vi "SParam VST Init.vi"(8 "error in":errorcluster, 11 "SPML Settings":T2={"VST Resource Name"="VNA-5633", "RFSG Port"="", "RFmx Port"="", "RF Out Switch"="VNA-5633", "RF Out Connection"={"Common RFout"="", "Port1 Incident"="", "Port2 Incident"=""}, "RF In Switch"="VNA-5633", "RF In Connection"={"Common RFin"="", "Port1 Reference"="", "Port1 Test"="", "Port2 Reference"="", "Port2 Test"=""}, "RFSG attenuation mode"=enum."Constant Attenuation", "RFSG Constant Attenuation (dB)"=0.0, "Save Calibration File at"=path "", "Short S1P"=path "", "Open S1P"=path "", "Load S1P"=path "", "Through Adapter S2P"=path ""}) -> (0 "error out":errorcluster, 3 "S-Par Reference Out":T1)   [LabVIEW 2023]
uses:
  Controls/Hardware Config - SParam_VST.ctl
  <vilib>/niSPML/Typedefs/Session Handle.ctl
  <vilib>/niSPML/S-Par Reference.lvclass
  FPT_SParam_Switching/Switch Configuration.ctl
  FPT_SParam_Switching/FPT_SParam_Switching.lvclass
  C:/Program Files/National Instruments/LabVIEW 2023/vi.lib/niSPML/Switching/2 Couplers Per Port 1 VST/S-Par 2 Couplers Per Port 1 VST Switching.lvclass
  <vilib>/niSPML/Configure Topology (2CperPort1VST).vi
  <vilib>/niSPML/S-Parameter Measurements.lvlib
  C:/Users/rfuser/Documents/srd-adg-rf/src/fpt/Alpha_Demo/S Param VST Test/FPT_SParam_VST/Measurement/FPT_SParam_Switching/FPT_SParam_Switching.lvclass
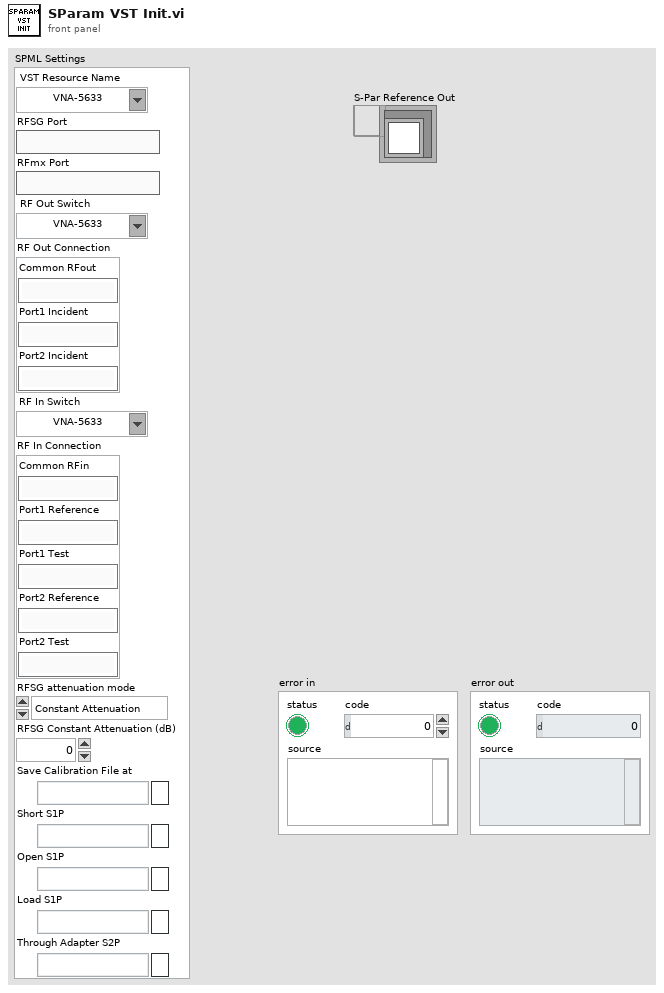
[diagram p1: front panel]
types:
  T1 = typedef "S-Parameter Measurements.lvlib/S-Par Reference.lvclass/Session Handle.ctl" = refnum<data-value>
  T2 = typedef "Hardware Config - SParam_VST.ctl" = cluster{"VST Resource Name":refnum<k15>, "RFSG Port":string, "RFmx Port":string, "RF Out Switch":refnum<k15>, "RF Out Connection":cluster{"Common RFout":string, "Port1 Incident":string, "Port2 Incident":string}, "RF In Switch":refnum<k15>, "RF In Connection":cluster{"Common RFin":string, "Port1 Reference":string, "Port1 Test":string, "Port2 Reference":string, "Port2 Test":string}, "RFSG attenuation mode":enum32{"<None>", "Constant Attenuation"}, "RFSG Constant Attenuation (dB)":dbl, "Save Calibration File at":path, "Short S1P":path, "Open S1P":path, "Load S1P":path, "Through Adapter S2P":path}
  T3 = typedef "FPT_SParam_Switching.lvclass/Switch Configuration.ctl" = cluster{"Common RFout":string, "Port1 Incident":string, "Port2 Incident":string, "Port1 Reference":string, "Port1 Test":string, "Common RFin":string, "Port2 Reference":string, "Port2 Test":string, "RF Out Switch":refnum<k15>, "RF In Switch":refnum<k15>}
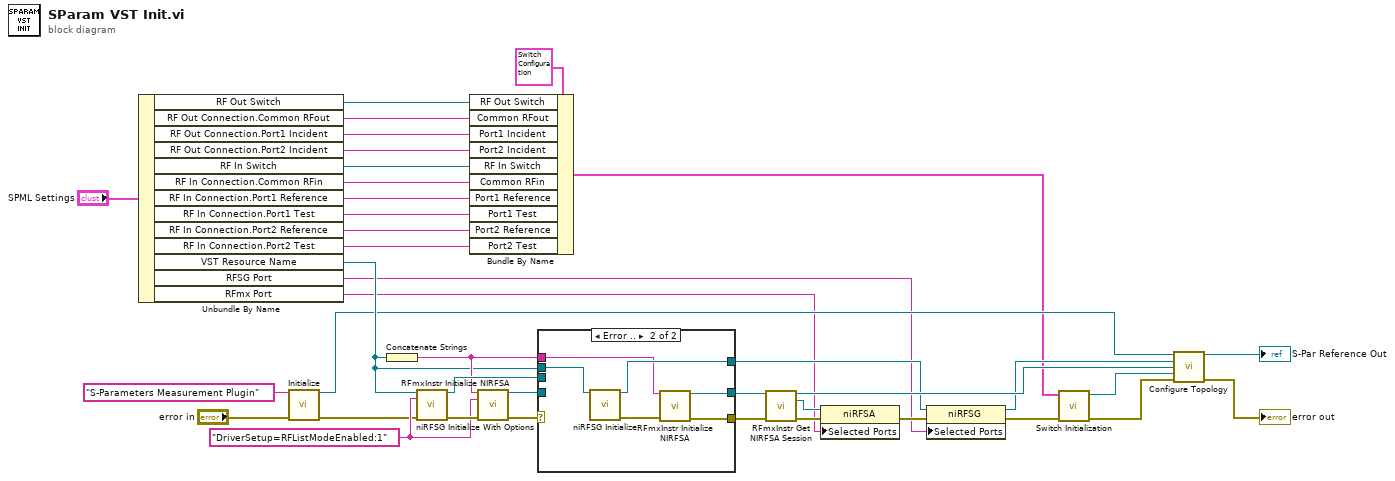
[diagram p0: block diagram]
diagram:
  w36 = "DriverSetup=RFListModeEnabled:1" ("option string")
  n1 = Unbundle By Name("SPML Settings") -> ("RF Out Switch"=w17:refnum<k15>, "RF Out Connection.Common RFout"=w18:string, "RF Out Connection.Port1 Incident"=w19:string, "RF Out Connection.Port2 Incident"=w21:string, "RF In Switch"=w20:refnum<k15>, "RF In Connection.Common RFin"=w22:string, "RF In Connection.Port1 Reference"=w23:string, "RF In Connection.Port1 Test"=w24:string, "RF In Connection.Port2 Reference"=w25:string, "RF In Connection.Port2 Test"=w26:string, "VST Resource Name"=w29:refnum<k15>, "RFSG Port"=w5:string, "RFmx Port"=w6:string)
  n2 = call <vilib>:"Initialize.vi"("Session Name"="S-Parameters Measurement Plugin", "error in"="error in") -> ("S-Par Reference Out"=w28:T1, "error out"=w31:errorcluster)  [unwired: 12 in]
  n3 = Concatenate Strings(w29) -> (w32:string)
  n4 = call <instrlib>:"niRFSG Initialize With Options.vi"("resource name"=w29, "option string"=w36, "error in"=w31) -> ("instrument handle"=w33:refnum<k15>, "error out"=w37:errorcluster)  [unwired: 11 in]
  n5 = Bundle By Name(cluster=T3 {"Common RFout"="PXI1Slot9", "Port1 Incident"="COM", "Port2 Incident"="CH1", "Port1 Reference"="CH2", "Port1 Test"="CH6", "Common RFin"="CH1", "Port2 Reference"="COM", "Port2 Test"="PXI1Slot12", "RF Out Switch"="CH5", "RF In Switch"="CH4"} ("Configurations"), "RF Out Switch"=w17, "Common RFout"=w18, "Port1 Incident"=w19, "Port2 Incident"=w21, "RF In Switch"=w20, "Common RFin"=w22, "Port1 Reference"=w23, "Port1 Test"=w24, "Port2 Reference"=w25, "Port2 Test"=w26) -> (w3:T3)
  n6 = call <vilib>:"RFmxInstr Initialize NIRFSA.vi"("Resource Name"=w32, "Option String"=w36, "error in (no error)"=w37) -> ("Instrument Handle Out"=w34:refnum<k21>, "error out"=w35:errorcluster)  [unwired: 10 in, 1 out]
  n7 = case shown="Error .." w35 {
    selector: w35 -> [w40 _]
    tunnel: [w42 w45] -> w13
    tunnel: w34 -> [w42 _]
    tunnel: [w41 w48] -> w8
    tunnel: w33 -> [w41 _]
    tunnel: w32 -> [_ w46]
    tunnel: [w40 w44] -> w14
    tunnel: w29 -> [_ w43]
    frame No Error {
    }
    frame Error {
      n8 = call <instrlib>:"niRFSG Initialize.vi"("resource name"=w43) -> ("instrument handle"=w48:refnum<k15>, "error out"=w47:errorcluster)  [unwired: 13 in]
      n9 = call <vilib>:"RFmxInstr Initialize NIRFSA.vi"("Resource Name"=w46, "error in (no error)"=w47) -> ("Instrument Handle Out"=w45:refnum<k21>, "error out"=w44:errorcluster)  [unwired: 11 in, 1 out]
    }
  }
  n10 = call <vilib>:"RFmxInstr Get NIRFSA Session.vi"("Instrument Handle In"=w13, "error in (no error)"=w14) -> ("Instrument Handle Out"=w10:refnum<k21>, "NI RFSA Session"=w11:refnum<k15>, "error out"=w12:errorcluster)  [unwired: 11 in]
  n11 = property class="niRFSA"(reference=w11, error in=w12, "Selected Ports"=w6) -> (error out=w9:errorcluster)  [unwired: 1 out]
  n12 = property class="niRFSG"(reference=w8, error in=w9, "Selected Ports"=w5) -> (reference out=w7:refnum<k15>, error out=w4:errorcluster)
  n13 = call "Switch Initialization.vi"("error in (no error)"=w4, "Configurations"=w3) -> ("error out"=w1:errorcluster, "SParam Switch Reference"=w2:refnum<data-value>)  [unwired: 8 in]
  n14 = call-poly <vilib>:"Configure Topology.vi"("S-Par Reference In"=w28, "NI RFSG Session"=w7, "NI RFmx Session"=w10, "Switch Reference"=w2, "error in"=w1) -> ("S-Par Reference Out"=→"S-Par Reference Out":T1, "error out"=→"error out":errorcluster)  [unwired: 9 in]
